vi "Post_Message-myRIO_App.vi"(8 "error in (no error)":errorcluster, 9 "message":string, 10 "Services Token":string) -> (0 "error out":errorcluster, 2 "response":string)   [LabVIEW 2015]
uses:
  <vilib>/httpClient/POSTBuffer.vi
  <vilib>/httpClient/LabVIEWHTTPClient.lvlib
panel:
  out "concatenated string":string
  out "headers":string
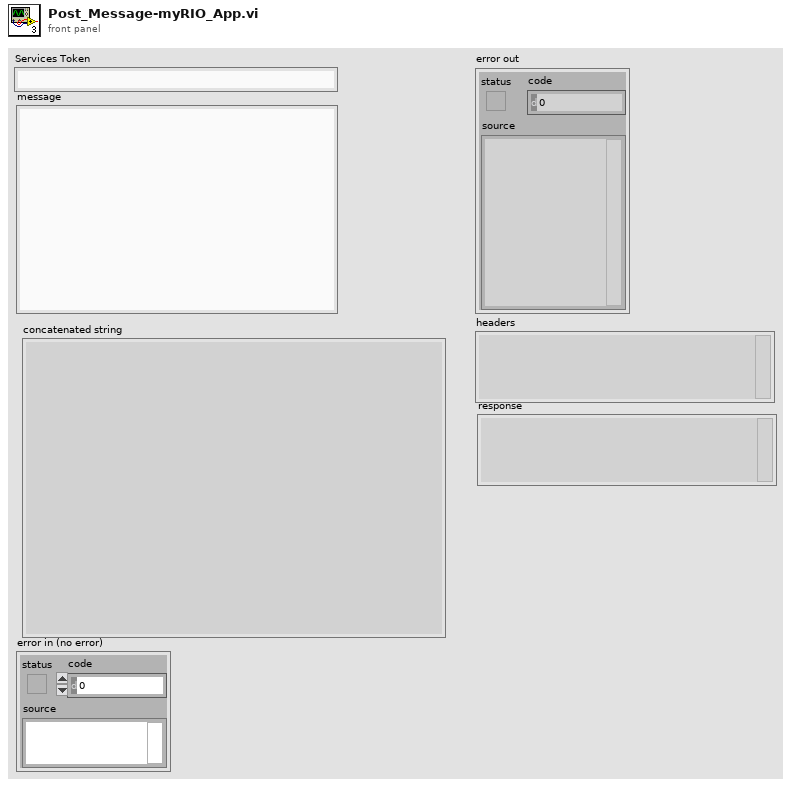
[diagram p1: front panel]
types:
  T1 = typedef "LabVIEWHTTPClient.lvlib/ClientHandle.ctl" = refnum<k1>
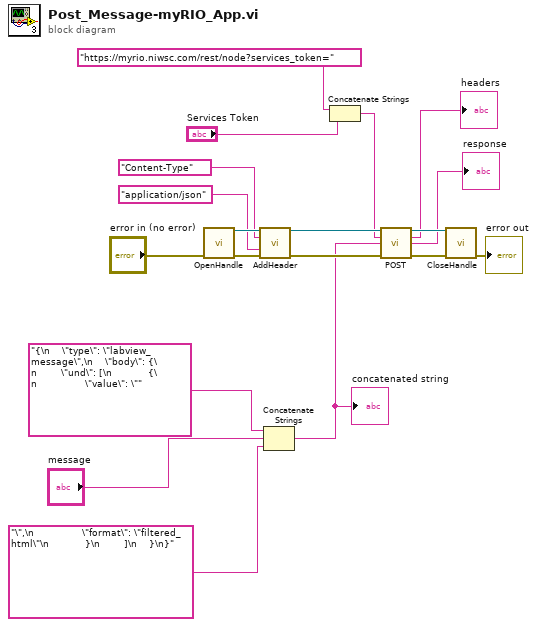
[diagram p0: block diagram]
diagram:
  n1 = call <vilib>:"OpenHandle.vi"("error in (no error)"="error in (no error)") -> ("client handle out"=w17:T1, "error out"=w16:errorcluster)  [unwired: 13 in]
  n2 = call <vilib>:"AddHeader.vi"("client handle"=w17, "header"="Content-Type", "value"="application/json", "error in (no error)"=w16) -> ("client handle out"=w12:T1, "error out"=w13:errorcluster)  [unwired: 10 in]
  n3 = Concatenate Strings("{\n    \"type\": \"labview_message\",\n    \"body\": {\n        \"und\": [\n            {\n                \"value\": \"" ("value"), "message", "\",\n                \"format\": \"filtered_html\"\n            }\n        ]\n    }\n}" ("value")) -> (w5:string)
  "concatenated string" <- w5
  n4 = Concatenate Strings("https://myrio.niwsc.com/rest/node?services_token=" ("value"), "Services Token") -> (w9:string)
  n5 = call-poly <vilib>:"POST.vi"("client handle"=w12, "url"=w9, "buffer"=w5, "error in (no error)"=w13) -> ("client handle out"=w18:T1, "headers"=→"headers":string, "body"=→"response":string, "error out"=w19:errorcluster)  [unwired: 8 in]
  n6 = call <vilib>:"CloseHandle.vi"("client handle"=w18, "error in (no error)"=w19) -> ("error out"=→"error out":errorcluster)  [unwired: 13 in]
